vi "Unified Leaf.vi"(7 "Actor in":refnum<class "Actor.lvclass">) -> (2 "Unified Leaf":bool)   [LabVIEW 2020, in "jettl.lvlib" / "Read Parent Attributes.lvlib"]
uses:
  Read Parent Attributes.lvlib
  Actor/Actor.lvclass
  Attributes/Attributes.lvclass
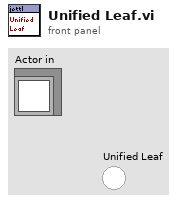
[diagram p1: front panel]
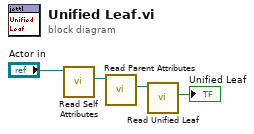
[diagram p0: block diagram]
diagram:
  n1 = call-dynamic "Read Self Attributes.vi"("Actor in"="Actor in") -> ("Self Attributes"=w4:refnum<class "Attributes.lvclass">)  [unwired: 10 in]
  n2 = call-dynamic "Read Parent Attributes.vi"("Attributes in"=w4) -> ("Parent Attributes"=w2:refnum<class "Attributes.lvclass">)  [unwired: 10 in]
  n3 = call-dynamic "Read Unified Leaf.vi"("Attributes in"=w2) -> ("Unified Leaf"=→"Unified Leaf":bool)  [unwired: 10 in]
